vi "Pre Launch Support.vi"(8 "error in":errorcluster, 11 "Manual UI in":refnum<class "Manual UI.lvclass">) -> (0 "error out":errorcluster, 3 "Manual UI out":refnum<class "Manual UI.lvclass">)   [LabVIEW 2019, in "Manual UI.lvlib" / "Manual UI.lvclass"]
uses:
  Project/Manual UI.lvclass
  C:/Users/Public/Documents/Development/builds/Engine/Engine.lvlibp/Project/Engine.lvclass
  Project/Manual UI.lvclass/Manual UI.ctl
  Accessors/Read Config.vi
  Accessors/Write Config.vi
  builds/Engine/Engine.lvlibp/Accessors/Read Directory.vi
  builds/Engine/Engine.lvlibp/Accessors/Write Change Instrument Event.vi
  builds/Tools/Config.lvlibp/Config.lvclass
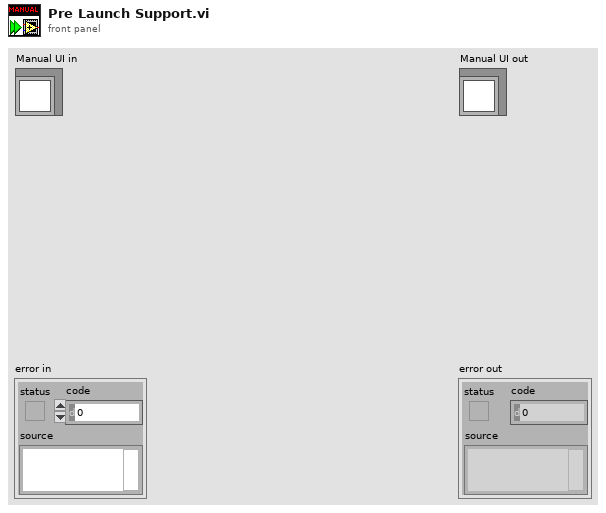
[diagram p1: front panel]
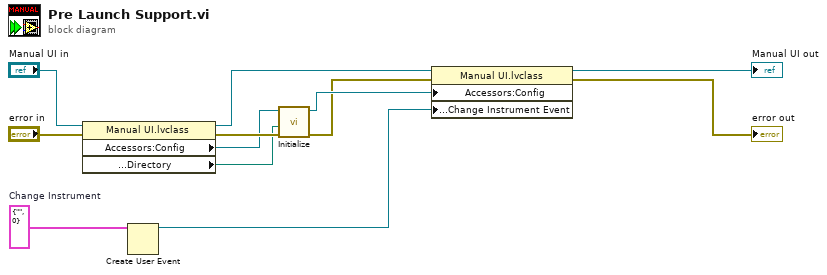
[diagram p0: block diagram]
diagram:
  w2 = cluster{"Identifier":string, "Panel":i32} {"Identifier"="", "Panel"=0}  # Change Instrument
  n1 = property class="Manual UI.lvclass"(reference="Manual UI in", error in="error in") -> (reference out=w6:refnum<class "Manual UI.lvclass">, error out=w10:errorcluster, "Accessors:Config"=w9:refnum<class "Config.lvclass">, "Accessors:Application:Information:Directory"=w8:path)
  n2 = Create User Event(user event datatype=w2) -> (user event=w1:refnum<user-event>)  [unwired: 1 in, 1 out]
  n3 = call-dynamic "Initialize.vi"("error in"=w10, "Path"=w8, "Config in"=w9) -> ("error out"=w3:errorcluster, "Config out"=w4:refnum<class "Config.lvclass">)  [unwired: 7 in]
  n4 = property class="Manual UI.lvclass"(reference=w6, error in=w3, "Accessors:Config"=w4, "Accessors:Events:Manual:Change Instrument Event"=w1) -> (reference out=→"Manual UI out":refnum<class "Manual UI.lvclass">, error out=→"error out":errorcluster)
